vi "PCO_SetFlimRelativePhase.vi"(8 "error in (no error)":errorcluster {"code" format="%x"}, 10 "dwPhaseMilliDeg":u32, 11 "ph":u64) -> (0 "error out":errorcluster {"code" format="%x"}, 2 "ErrorMessage":i32 format="%x", 3 "ph out":u64)   [LabVIEW 2020, in "SDK.lvlib" / "SpecialCommandsFlim.lvlib"]
doc: "<b>Description:</b>\nThis function does set the relative phase value, if the camera is configured for manual phase shifting (see function PCO_SetFlimPhaseSequenceParameter). No PCO_ArmCamera is required to change the relative phase setting, but the relative phase value is reset to zero, when the current mode is set to [manual shifting] and a PCO_ArmCamera is performed.\n\n<b>Supported camera type:</b>\npco.flim\n\n<b>Descriptor dependency:</b>\nNone"
uses:
  SpecialCommandsFlim.lvlib
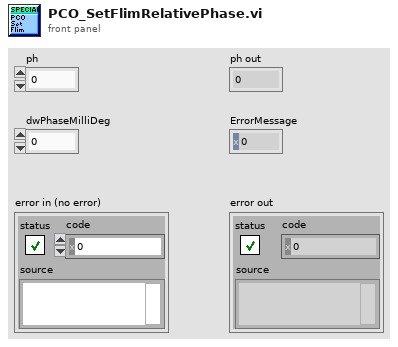
[diagram p1: front panel]
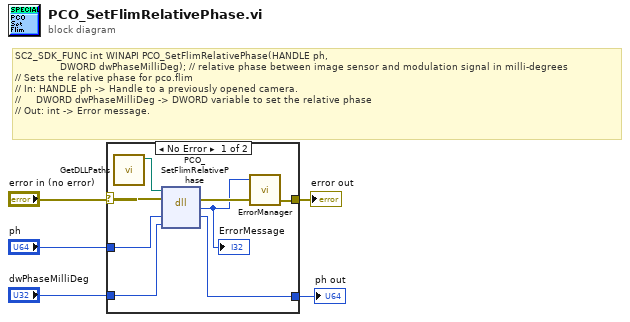
[diagram p0: block diagram]
diagram:
  # "SC2_SDK_FUNC int WINAPI PCO_SetFlimRelativePhase(HANDLE ph, \n               DWORD dwPhaseMilliDeg); // relative phase between image sensor and modulation signal in milli-degrees\n// Sets the relative phase for pco.flim\n// In: HANDLE ph -> Handle to a previously opened camera.\n//     DWORD dwPhaseMilliDeg -> DWORD variable to set the relative phase\n// Out: int -> Error message."
  n1 = case shown="No Error" "error in (no error)" {
    selector: "error in (no error)" -> [w10 w15]
    tunnel: "ph" -> [w13 w14]
    tunnel: [w12 w14] -> w4
    tunnel: "dwPhaseMilliDeg" -> [w11 _]
    tunnel: [w9 w15] -> w2
    frame No Error {
      n2 = call "GetDLLPaths.vi"() -> ("SC2_Cam_Path"=w6:path)  [unwired: 9 in, 2 out]
      n3 = dll-call lib="?" fn="PCO_SetFlimRelativePhase"(path in=w6, error in=w10, "ph"=w13, "dwPhaseMilliDeg"=w11) -> (error out=w8:errorcluster, "return type"=w7:i32, "ph"=w12:u64)  [unwired: 2 in, 1 out]
      "ErrorMessage" <- w7
      n4 = call "ErrorManager.vi"("error in (no error)"=w8, "error code"=w7) -> ("error out"=w9:errorcluster)  [unwired: 3 in]
    }
    frame Error {
    }
  }
  "ph out" <- w4
  "error out" <- w2
